vi "Display Package List.vi"() -> ()   [LabVIEW 2017, in "GCentral API.lvlib"]
uses:
  GCentral API.lvlib
  Package/Package.lvclass/Package.ctl
  Package/Read name.vi
  Package/Read description.vi
  Package/Read downloads.vi
  Package/Package.lvclass
panel:
  in  "Multicolumn Listbox":i32(listbox)
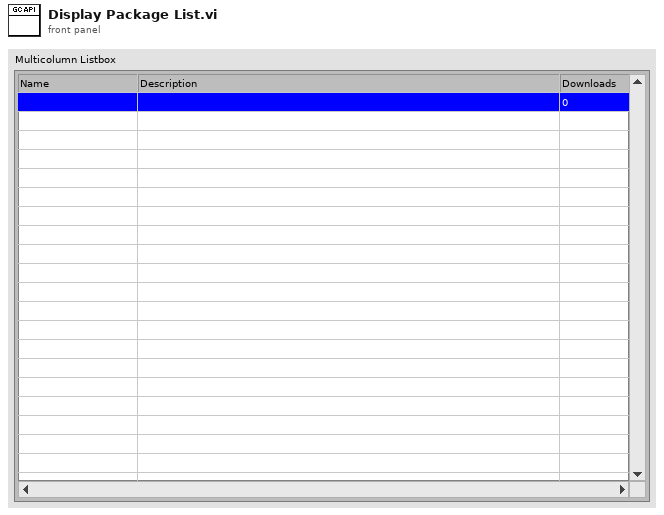
[diagram p1: front panel]
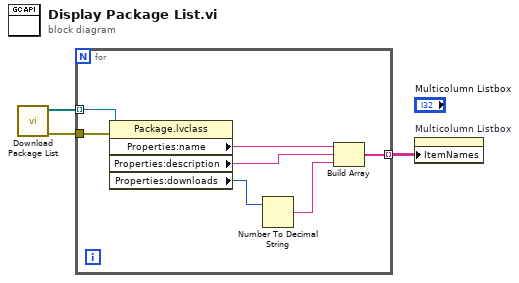
[diagram p0: block diagram]
diagram:
  n1 = call "Download Package List.vi"() -> ("error out"=w2:errorcluster, "Packages"=w3:refnum<class "Package.lvclass">[])  [unwired: 10 in]
  n2 = for {
    tunnel: w3 -> [w9] mode=indexing
    tunnel: w2 -> [w10]
    tunnel: [w4] -> w1 mode=indexing
    n3 = property class="Package.lvclass"(reference=w9, error in=w10) -> ("Properties:name"=w7:string, "Properties:description"=w6:string, "Properties:downloads"=w8:i32)  [unwired: 2 out]
    n4 = Number To Decimal String(number=w8) -> (decimal integer string=w5:string)  [unwired: 1 in]
    n5 = Build Array(w7, w6, w5) -> (w4:string[])
  }
  n6 = property on="Multicolumn Listbox" class="MCListbox (strict)"("ItemNames"=w1) -> ()  [unwired: 2 in, 2 out]
